vi "Write Instantiated by ref_.vi"(8 "error in (no error)":errorcluster, 10 "Instantiated by ref?":bool, 11 "LV RT in":refnum<class "LV RT.lvclass">) -> (0 "error out":errorcluster, 3 "LV RT out":refnum<class "LV RT.lvclass">)   [LabVIEW 2016, in "LV RT.lvclass"]
uses:
  LV RT.lvclass
  LV RT.lvclass/LV RT.ctl
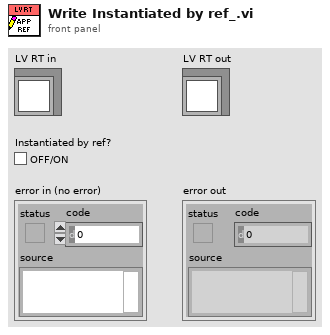
[diagram p1: front panel]
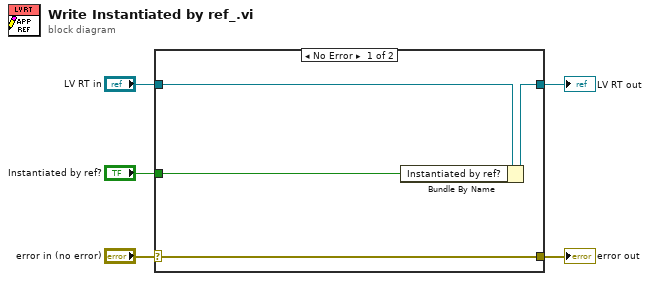
[diagram p0: block diagram]
diagram:
  n1 = case shown="No Error" "error in (no error)" {
    selector: "error in (no error)" -> [w9 w10]
    tunnel: [w9 w10] -> w4
    tunnel: [w7 w11] -> w2
    tunnel: "LV RT in" -> [w8 w11]
    tunnel: "Instantiated by ref?" -> [w6 _]
    frame No Error {
      n2 = Bundle By Name(cluster=w8, "Instantiated by ref?"=w6) -> (w7:refnum<class "LV RT.lvclass">)
    }
    frame Error {
    }
  }
  "error out" <- w4
  "LV RT out" <- w2
